vi "py-lv-comm_labview-client.vi"() -> ()   [LabVIEW 2013]
panel:
  in  "Update Time (ms)":i32=100
  out "Status":string="Idle"
  in  "Tab Control":enum32{"Python Communication", "Debug"}(tab)
  in  "Connect to Server":bool
  in  "Send Command":bool
  in  "Command":string
  in  "Wait for response":bool=TRUE
  in  "TCP address":string="tcp://127.0.0.1:5555" caption="TCP address of ZMQ server"
  out "Return string":string
  in  "Read Integer":bool
  in  "Read Double":bool
  in  "Read String":bool
  in  "Read Bool":bool
  in  "Read Numpy Array":bool
  in  "Function":string
  in  "Python Property":bool=TRUE
  in  "Arguments":string[](array[string])
  out "int result":i32
  out "double result":dbl
  out "string result":string
  out "bool result":bool
  out "nparray result":dbl[](array[numeric])
  out "error":errorcluster
  out "Overload":bool
  out "# elements in queue":i32
  in  "stop":bool
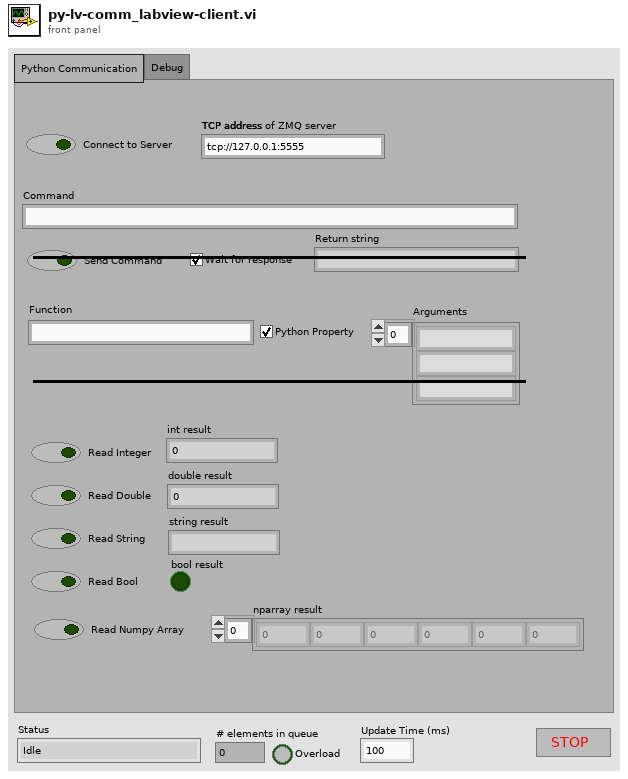
[diagram p1: front panel]
types:
  T1 = cluster{"zmq_context out":refnum<class "zmq_context.lvclass">, "socket out":refnum<class "zmq_socket.lvclass">}
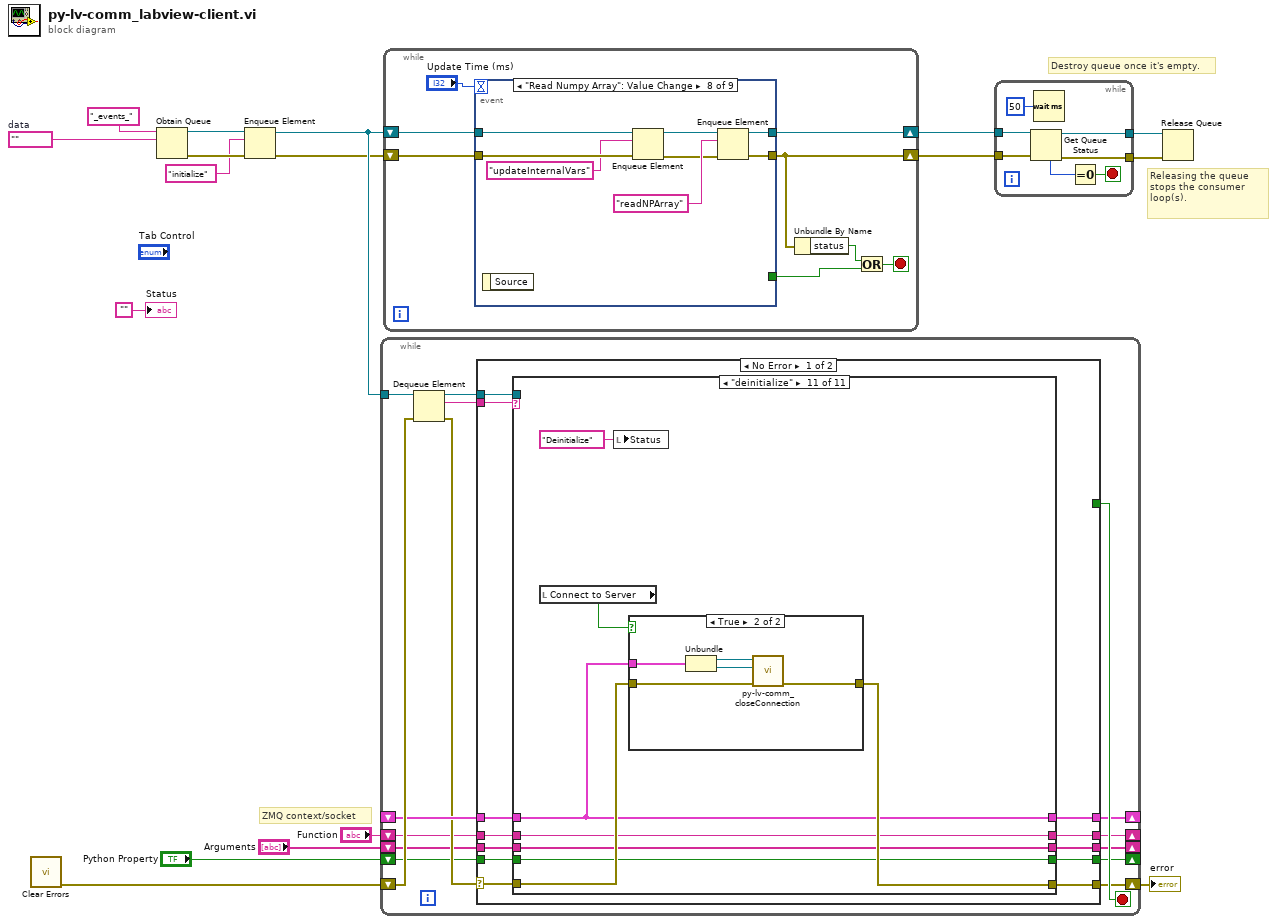
[diagram p0: block diagram]
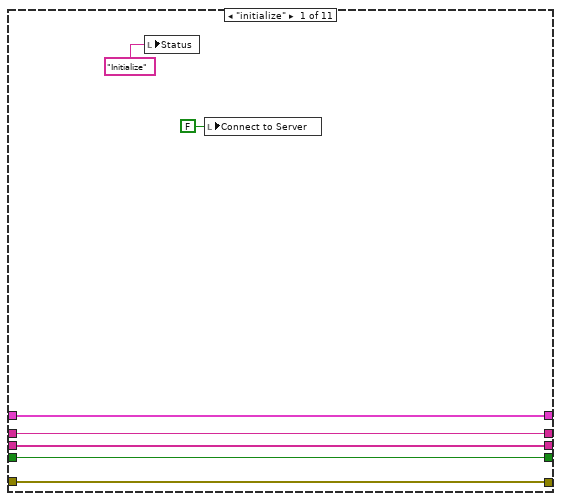
[diagram p2: hidden frame]
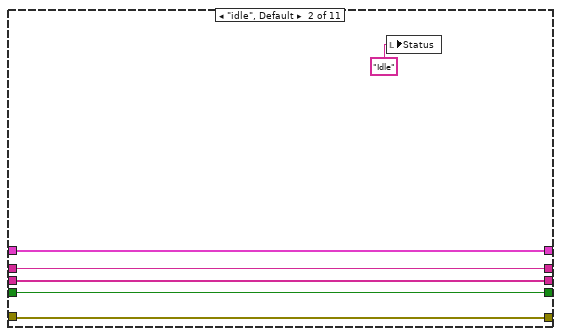
[diagram p3: hidden frame]
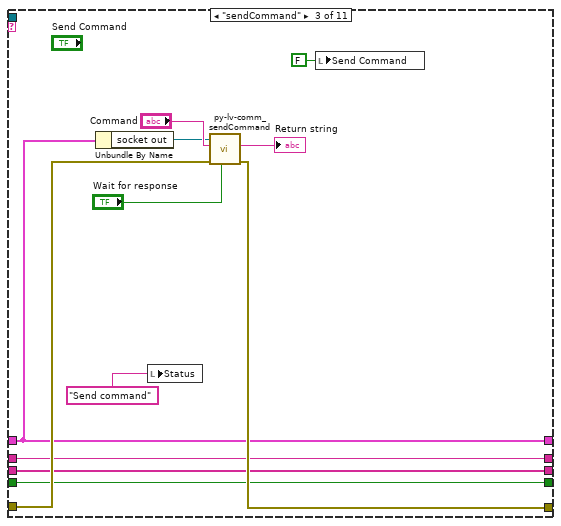
[diagram p4: hidden frame]
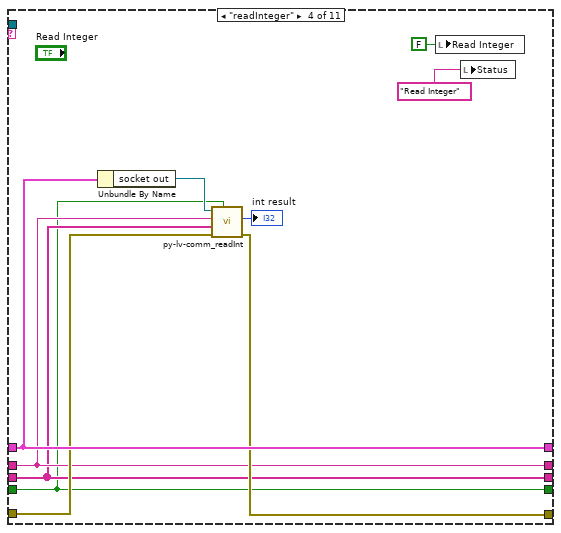
[diagram p5: hidden frame]
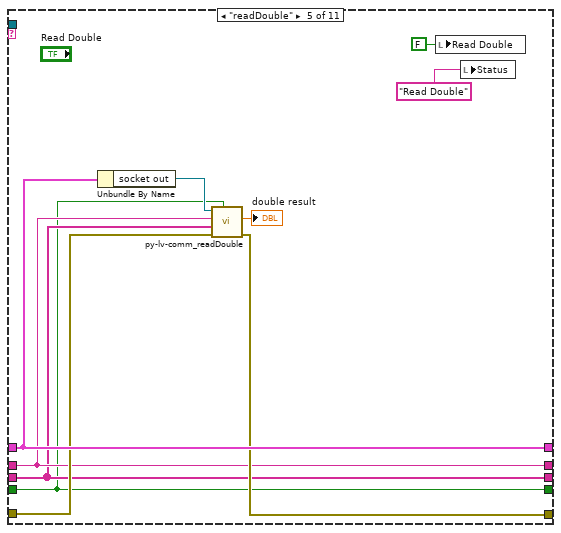
[diagram p6: hidden frame]
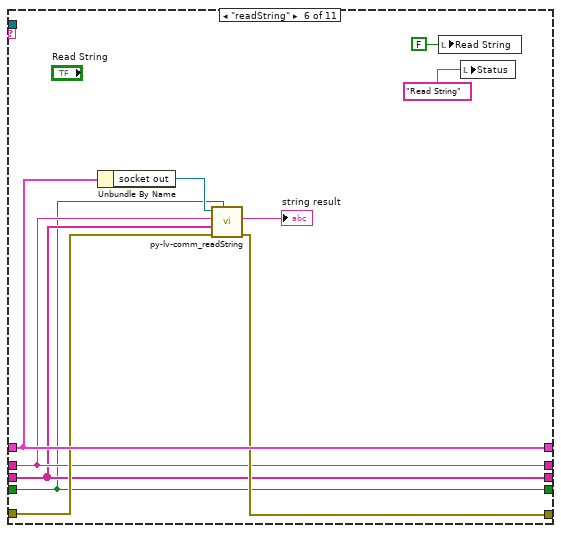
[diagram p7: hidden frame]
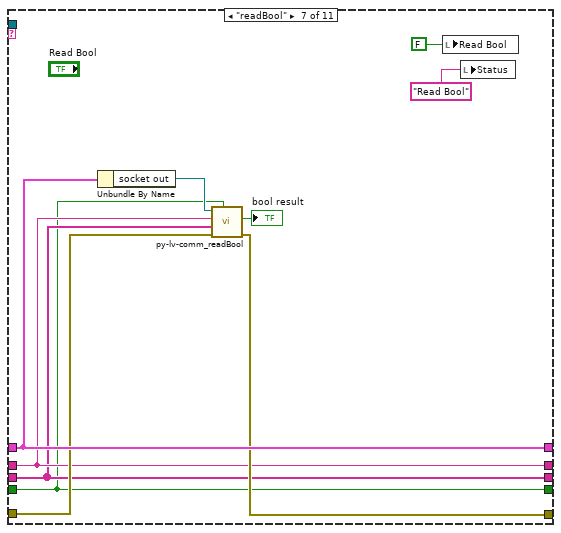
[diagram p8: hidden frame]
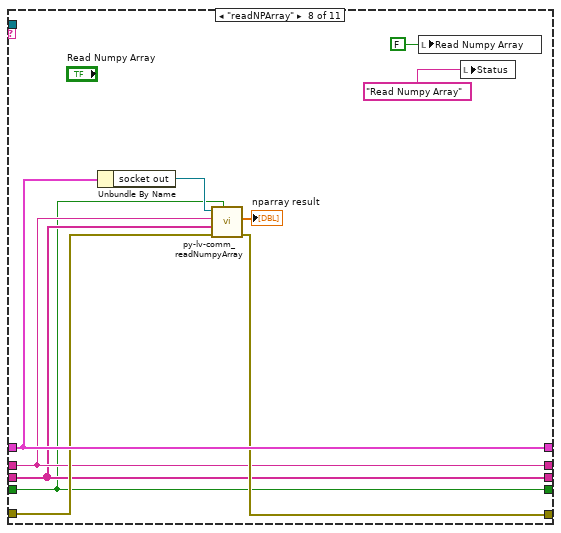
[diagram p9: hidden frame]
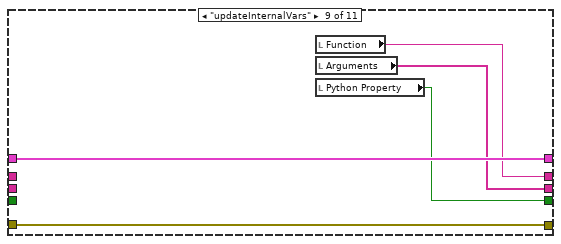
[diagram p10: hidden frame]
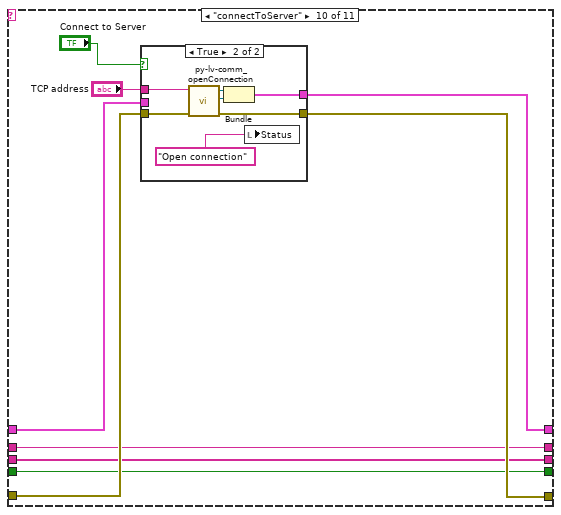
[diagram p11: hidden frame]
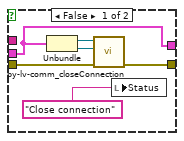
[diagram p12: hidden frame]
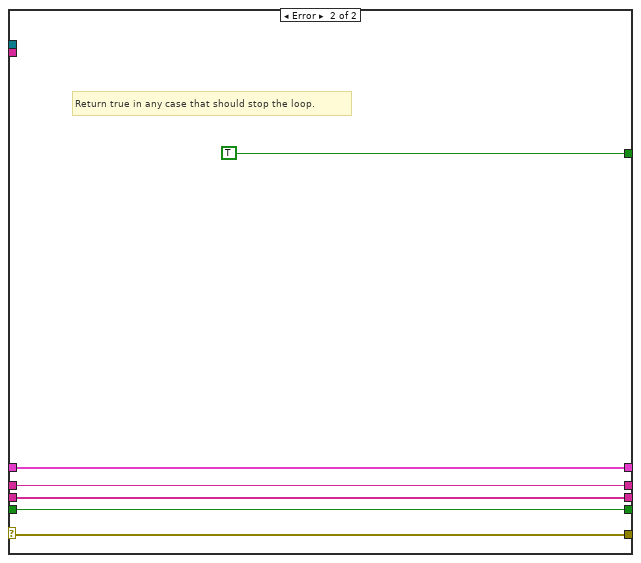
[diagram p14: hidden frame]
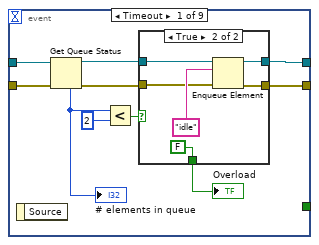
[diagram p15: hidden frame]
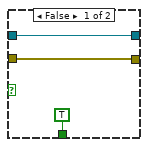
[diagram p16: hidden frame]
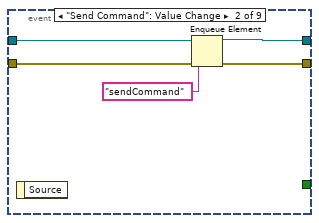
[diagram p17: hidden frame]
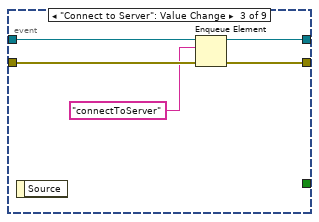
[diagram p18: hidden frame]
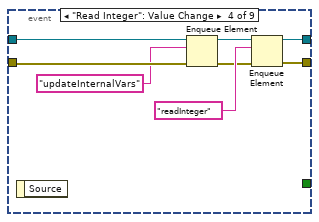
[diagram p19: hidden frame]
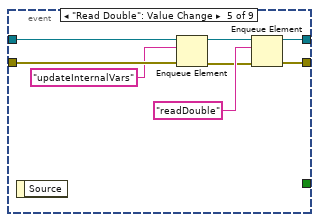
[diagram p20: hidden frame]
diagram:
  w17 = ""  # data
  # "ZMQ context/socket"
  # "Destroy queue once it's empty."
  # "Releasing the queue stops the consumer loop(s)."
  n1 = call <vilib>:"Clear Errors.vi"() -> ("error out"=w7:errorcluster)  [unwired: 7 in]
  n2 = Obtain Queue(name (unnamed)="_events_", element data type=w17) -> (queue out=w13:refnum<queue>, error out=w12:errorcluster)  [unwired: 3 in, 1 out]
  n3 = Enqueue Element(queue=w13, element="initialize", error in (no error)=w12) -> (queue out=w11:refnum<queue>, error out=w10:errorcluster)  [unwired: 1 in, 1 out]
  n4 = while {
    tunnel: w11 -> [w32]
    shift-right: [w26] -> w4
    shift-left: w7 -> [w29]
    shift-right: [w28] -> _
    shift-left: _ -> [w27]
    shift-right: [w20] -> _
    shift-left: "Function" -> [w23]
    shift-right: [w19] -> _
    shift-left: "Arguments" -> [w22]
    shift-right: [w18] -> _
    shift-left: "Python Property" -> [w21]
    stop <- w30 stop-if-true
    n5 = Dequeue Element(queue=w32, error in (no error)=w29) -> (queue out=w24:refnum<queue>, element=w31:string, error out=w25:errorcluster)  [unwired: 1 in, 1 out]
    n6 = case shown="No Error" w25 {
      selector: w25 -> [w43 w164]
      tunnel: w31 -> [w44 _]
      tunnel: [_ TRUE] -> w30
      tunnel: [w42 w165] -> w28
      tunnel: w27 -> [w41 w165]
      tunnel: [w40 w164] -> w26
      tunnel: w24 -> [w39 _]
      tunnel: w23 -> [w38 w163]
      tunnel: w22 -> [w37 w162]
      tunnel: w21 -> [w36 w161]
      tunnel: [w35 w163] -> w20
      tunnel: [w34 w162] -> w19
      tunnel: [w33 w161] -> w18
      frame No Error {
        n7 = case shown="\"deinitialize\"" w44 {
          tunnel: w43 -> [w49 w52 w69 w75 w85 w95 w105 w115 w123 w131 w153]
          tunnel: [w50 w56 w65 w76 w86 w96 w106 w116 w124 w130 w151] -> w42
          tunnel: w41 -> [w50 w56 w65 w76 w86 w96 w106 w116 w124 w129 w151]
          tunnel: [w49 w52 w66 w74 w84 w94 w104 w114 w123 w128 w152] -> w40
          tunnel: w39 -> [_ _ _ _ _ _ _ _ _ _ _]
          tunnel: w38 -> [w47 w55 w60 w72 w82 w92 w102 w112 _ w127 w150]
          tunnel: w37 -> [w46 w54 w59 w71 w81 w91 w101 w111 _ w126 w149]
          tunnel: w36 -> [w45 w53 w58 w70 w80 w90 w100 w110 _ w125 w148]
          tunnel: [w47 w55 w60 w72 w82 w92 w102 w112 w122 w127 w150] -> w35
          tunnel: [w46 w54 w59 w71 w81 w91 w101 w111 w121 w126 w149] -> w34
          tunnel: [w45 w53 w58 w70 w80 w90 w100 w110 w120 w125 w148] -> w33
          frame "initialize" {
            n8 = local write "Status"("Initialize" ("Status")) -> ()
            n9 = local write "Connect to Server"(FALSE ("Connect to Server")) -> ()
          }
          frame "idle", Default {
            n10 = local write "Status"("Idle" ("Status")) -> ()
          }
          frame "sendCommand" {
            n11 = Unbundle By Name(w65) -> ("socket out"=w63:refnum<class "zmq_socket.lvclass">)
            n12 = local write "Status"("Send command" ("Status")) -> ()
            n13 = call "py-lv-comm_sendCommand.vi"("Wait for response (T)"="Wait for response", "error in (no error)"=w69, "command"="Command", "zmq_socket in"=w63) -> ("error out"=w66:errorcluster, "data"=→"Return string":string)  [unwired: 5 in, 1 out]
            n14 = local write "Send Command"(FALSE ("Send Command")) -> ()
          }
          frame "readInteger" {
            n15 = Unbundle By Name(w76) -> ("socket out"=w77:refnum<class "zmq_socket.lvclass">)
            n16 = call "py-lv-comm_readInt.vi"("Property"=w70, "error in (no error)"=w75, "arguments"=w71, "function"=w72, "zmq_socket in"=w77) -> ("error out"=w74:errorcluster, "int result"=→"int result":i32)  [unwired: 4 in, 1 out]
            n17 = local write "Read Integer"(FALSE ("Read Integer")) -> ()
            n18 = local write "Status"("Read Integer" ("Status")) -> ()
          }
          frame "readDouble" {
            n19 = Unbundle By Name(w86) -> ("socket out"=w87:refnum<class "zmq_socket.lvclass">)
            n20 = call "py-lv-comm_readDouble.vi"("Property"=w80, "error in (no error)"=w85, "arguments"=w81, "function"=w82, "zmq_socket in"=w87) -> ("error out"=w84:errorcluster, "double result"=→"double result":dbl)  [unwired: 4 in, 1 out]
            n21 = local write "Read Double"(FALSE ("Read Integer")) -> ()
            n22 = local write "Status"("Read Double" ("Status")) -> ()
          }
          frame "readString" {
            n23 = Unbundle By Name(w96) -> ("socket out"=w97:refnum<class "zmq_socket.lvclass">)
            n24 = call "py-lv-comm_readString.vi"("Property"=w90, "error in (no error)"=w95, "arguments"=w91, "function"=w92, "zmq_socket in"=w97) -> ("error out"=w94:errorcluster, "string result"=→"string result":string)  [unwired: 4 in, 1 out]
            n25 = local write "Read String"(FALSE ("Read Integer")) -> ()
            n26 = local write "Status"("Read String" ("Status")) -> ()
          }
          frame "readBool" {
            n27 = Unbundle By Name(w106) -> ("socket out"=w107:refnum<class "zmq_socket.lvclass">)
            n28 = call "py-lv-comm_readBool.vi"("Property"=w100, "error in (no error)"=w105, "arguments"=w101, "function"=w102, "zmq_socket in"=w107) -> ("error out"=w104:errorcluster, "bool result"=→"bool result":bool)  [unwired: 4 in, 1 out]
            n29 = local write "Read Bool"(FALSE ("Read Integer")) -> ()
            n30 = local write "Status"("Read Bool" ("Status")) -> ()
          }
          frame "readNPArray" {
            n31 = Unbundle By Name(w116) -> ("socket out"=w117:refnum<class "zmq_socket.lvclass">)
            n32 = call "py-lv-comm_readNumpyArray.vi"("Property"=w110, "error in (no error)"=w115, "arguments"=w111, "function"=w112, "zmq_socket in"=w117) -> ("error out"=w114:errorcluster, "nparray result"=→"nparray result":dbl[])  [unwired: 4 in, 1 out]
            n33 = local write "Read Numpy Array"(FALSE ("Read Integer")) -> ()
            n34 = local write "Status"("Read Numpy Array" ("Status")) -> ()
          }
          frame "updateInternalVars" {
            n35 = local read "Function"() -> (w122:string)
            n36 = local read "Arguments"() -> (w121:string[])
            n37 = local read "Python Property"() -> (w120:bool)
          }
          frame "connectToServer" {
            n38 = case shown="True" "Connect to Server" {
              tunnel: "TCP address" -> [_ w146]
              tunnel: w131 -> [w139 w145]
              tunnel: [w138 w144] -> w128
              tunnel: [w135 w141] -> w130
              tunnel: w129 -> [w135 _]
              frame False {
                n39 = Unbundle(w135) -> ("zmq_context out"=w137:refnum<class "zmq_context.lvclass">, "socket out"=w136:refnum<class "zmq_socket.lvclass">)
                n40 = call "py-lv-comm_closeConnection.vi"("error in (no error)"=w139, "socket in"=w136, "zmq_context in"=w137) -> ("error out"=w138:errorcluster)  [unwired: 8 in]
                n41 = local write "Status"("Close connection" ("Status")) -> ()
              }
              frame True {
                n42 = call "py-lv-comm_openConnection.vi"("error in"=w145, "TCP address"=w146) -> ("error out"=w144:errorcluster, "socket out"=w142:refnum<class "zmq_socket.lvclass">, "zmq_context out"=w143:refnum<class "zmq_context.lvclass">)  [unwired: 7 in]
                n43 = Bundle("zmq_context out"=w143, "socket out"=w142) -> (w141:T1)  [unwired: 1 in]
                n44 = local write "Status"("Open connection" ("Status")) -> ()
              }
            }
          }
          frame "deinitialize" {
            n45 = local read "Connect to Server"() -> (w147:bool)
            n46 = local write "Status"("Deinitialize" ("Status")) -> ()
            n47 = case shown="True" w147 {
              tunnel: w153 -> [w155 w158]
              tunnel: [w155 w157] -> w152
              tunnel: w151 -> [_ w156]
              frame False {
              }
              frame True {
                n48 = Unbundle(w156) -> ("zmq_context out"=w160:refnum<class "zmq_context.lvclass">, "socket out"=w159:refnum<class "zmq_socket.lvclass">)
                n49 = call "py-lv-comm_closeConnection.vi"("error in (no error)"=w158, "socket in"=w159, "zmq_context in"=w160) -> ("error out"=w157:errorcluster)  [unwired: 8 in]
              }
            }
          }
        }
      }
      frame Error {
        # "Return true in any case that should stop the loop."
      }
    }
  }
  "error" <- w4
  n50 = while {
    shift-right: [w167] -> w6
    shift-left: w10 -> [w169]
    shift-right: [w168] -> w5
    shift-left: w11 -> [w174]
    stop <- w172 stop-if-true
    n51 = event shown="[7] \"Read Numpy Array\": Value Change" {
      selector: _ -> [_ _ _ _ _ _ _ _ _]
      dyn-events: _ -> [_ _ _ _ _ _ _ _ _]
      timeout: "Update Time (ms)" -> [_ _ _ _ _ _ _ _ _]
      tunnel: w174 -> [w178 w198 w203 w206 w214 w222 w232 w240 w248]
      tunnel: w169 -> [w177 w196 w202 w205 w213 w221 w230 w239 w247]
      tunnel: [w182 w195 w200 w210 w218 w226 w234 w242 w246] -> w167
      tunnel: [_ _ _ _ _ _ _ _ "stop"] -> w173
      tunnel: [w179 w197 w199 w209 w217 w225 w233 w241 w245] -> w168
      event Timeout {
        n52 = event-data() -> ()  [unwired: 1 in, 1 out]
        n53 = Get Queue Status(queue=w178, error in (no error)=w177) -> (queue out=w175:refnum<queue>, error out=w176:errorcluster, # elements in queue=w183:i32)  [unwired: 1 in, 5 out]
        "# elements in queue" <- w183
        n54 = Less?(x=w183, y=2) -> (x < y?=w180:bool)
        n55 = case shown="True" w180 {
          tunnel: [w186 w192] -> w179
          tunnel: [w185 w191] -> w182
          tunnel: [TRUE ("Overload") FALSE ("Overload")] -> w181
          tunnel: w175 -> [w186 w188]
          tunnel: w176 -> [w185 w189]
          frame False {
          }
          frame True {
            n56 = Enqueue Element(queue=w188, element="idle", error in (no error)=w189) -> (queue out=w192:refnum<queue>, error out=w191:errorcluster)  [unwired: 1 in, 1 out]
          }
        }
        "Overload" <- w181
      }
      event "Send Command": Value Change {
        n57 = event-data() -> ()  [unwired: 1 in, 1 out]
        n58 = Enqueue Element(queue=w198, element="sendCommand", error in (no error)=w196) -> (queue out=w197:refnum<queue>, error out=w195:errorcluster)  [unwired: 1 in, 1 out]
      }
      event "Connect to Server": Value Change {
        n59 = event-data() -> ()  [unwired: 1 in, 1 out]
        n60 = Enqueue Element(queue=w203, element="connectToServer", error in (no error)=w202) -> (queue out=w199:refnum<queue>, error out=w200:errorcluster)  [unwired: 1 in, 1 out]
      }
      event "Read Integer": Value Change {
        n61 = event-data() -> ()  [unwired: 1 in, 1 out]
        n62 = Enqueue Element(queue=w206, element="updateInternalVars", error in (no error)=w205) -> (queue out=w208:refnum<queue>, error out=w207:errorcluster)  [unwired: 1 in, 1 out]
        n63 = Enqueue Element(queue=w208, element="readInteger", error in (no error)=w207) -> (queue out=w209:refnum<queue>, error out=w210:errorcluster)  [unwired: 1 in, 1 out]
      }
      event "Read Double": Value Change {
        n64 = event-data() -> ()  [unwired: 1 in, 1 out]
        n65 = Enqueue Element(queue=w214, element="updateInternalVars", error in (no error)=w213) -> (queue out=w216:refnum<queue>, error out=w215:errorcluster)  [unwired: 1 in, 1 out]
        n66 = Enqueue Element(queue=w216, element="readDouble", error in (no error)=w215) -> (queue out=w217:refnum<queue>, error out=w218:errorcluster)  [unwired: 1 in, 1 out]
      }
      event "Read String": Value Change {
        n67 = event-data() -> ()  [unwired: 1 in, 1 out]
        n68 = Enqueue Element(queue=w222, element="updateInternalVars", error in (no error)=w221) -> (queue out=w224:refnum<queue>, error out=w223:errorcluster)  [unwired: 1 in, 1 out]
        n69 = Enqueue Element(queue=w224, element="readString", error in (no error)=w223) -> (queue out=w225:refnum<queue>, error out=w226:errorcluster)  [unwired: 1 in, 1 out]
      }
      event "Read Bool": Value Change {
        n70 = event-data() -> ()  [unwired: 1 in, 1 out]
        n71 = Enqueue Element(queue=w232, element="updateInternalVars", error in (no error)=w230) -> (queue out=w231:refnum<queue>, error out=w228:errorcluster)  [unwired: 1 in, 1 out]
        n72 = Enqueue Element(queue=w231, element="readBool", error in (no error)=w228) -> (queue out=w233:refnum<queue>, error out=w234:errorcluster)  [unwired: 1 in, 1 out]
      }
      event "Read Numpy Array": Value Change {
        n73 = event-data() -> ()  [unwired: 1 in, 1 out]
        n74 = Enqueue Element(queue=w240, element="updateInternalVars", error in (no error)=w239) -> (queue out=w237:refnum<queue>, error out=w238:errorcluster)  [unwired: 1 in, 1 out]
        n75 = Enqueue Element(queue=w237, element="readNPArray", error in (no error)=w238) -> (queue out=w241:refnum<queue>, error out=w242:errorcluster)  [unwired: 1 in, 1 out]
      }
      event "stop": Value Change {
        n76 = event-data() -> ()  [unwired: 1 in, 1 out]
        n77 = Enqueue Element(queue=w248, element="deinitialize", error in (no error)=w247) -> (queue out=w245:refnum<queue>, error out=w246:errorcluster)  [unwired: 1 in, 1 out]
      }
    }
    n78 = Unbundle By Name(w167) -> ("status"=w171:bool)
    n79 = Or(x=w171, y=w173) -> (x .or. y?=w172:bool)
  }
  n80 = while {
    tunnel: [w255] -> w14
    tunnel: [w252] -> w15
    tunnel: w6 -> [w251]
    tunnel: w5 -> [w250]
    stop <- w253 stop-if-true
    n81 = Get Queue Status(queue=w250, error in (no error)=w251) -> (queue out=w252:refnum<queue>, error out=w255:errorcluster, # elements in queue=w254:i32)  [unwired: 1 in, 5 out]
    n82 = Wait (ms)(milliseconds to wait=u32 50) -> ()  [unwired: 1 out]
    n83 = Equal To 0?(x=w254) -> (x = 0?=w253:bool)
  }
  n84 = Release Queue(queue=w15, error in (no error)=w14) -> ()  [unwired: 1 in, 3 out]
  "Status" <- ""
